vi "Parse Config Data.vi"(8 "error in (no error)":errorcluster, 10 "Custom Config Data":u8[](array[numeric]), 11 "CIFfifo in":refnum<class "CIFfifo.lvclass">) -> (0 "error out":errorcluster, 2 "Depth":u64, 3 "CIFfifo out":refnum<class "CIFfifo.lvclass">)   [LabVIEW 2021, in "CIFfifo.lvclass"]
uses:
  CIFfifo.lvclass
  CIFfifo.lvclass/CIFfifo.ctl
  Accessors/Write Flags.vi
  Utilities/Expand FIFO Flags.vi
  ChannelCommon.lvlib
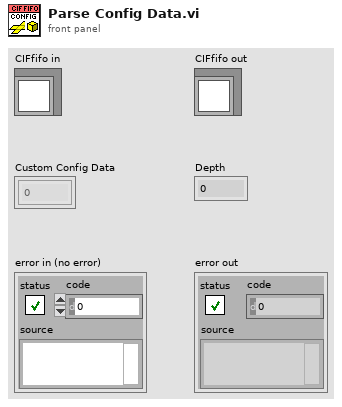
[diagram p1: front panel]
types:
  T1 = typedef "ChannelCommon.lvlib/FIFO Config.ctl" = cluster{"Depth":u64, "Flags":u64}
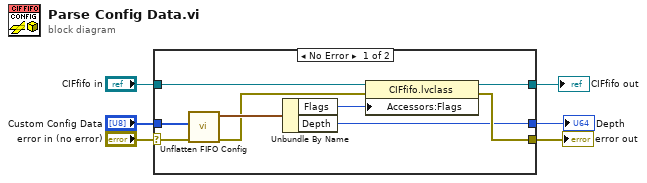
[diagram p0: block diagram]
diagram:
  n1 = case shown="No Error" "error in (no error)" {
    selector: "error in (no error)" -> [w10 w17]
    tunnel: [w9 w17] -> w5
    tunnel: [w13 w16] -> w3
    tunnel: "CIFfifo in" -> [w7 w16]
    tunnel: "Custom Config Data" -> [w12 _]
    tunnel: [w8 _] -> w1
    frame No Error {
      n2 = call "Unflatten FIFO Config.vi"("error in"=w10, "Flattened Data in"=w12) -> ("error out"=w11:errorcluster, "FIFO Config out"=w15:T1)  [unwired: 7 in, 1 out]
      n3 = Unbundle By Name(w15) -> ("Flags"=w14:u64, "Depth"=w8:u64)
      n4 = property class="CIFfifo.lvclass"(reference=w7, error in=w11, "Accessors:Flags"=w14) -> (reference out=w13:refnum<class "CIFfifo.lvclass">, error out=w9:errorcluster)
    }
    frame Error {
    }
  }
  "error out" <- w5
  "CIFfifo out" <- w3
  "Depth" <- w1
